vi "Example.vi"() -> ()   [LabVIEW 2019, in "BlueSerializationExample.lvlib"]
uses:
  BlueSerializationExample.lvlib
  BlueSerializable/BlueSerializable.lvclass
  BlueSerializer/BlueSerializer.lvclass
  2a9530f9-e359-4f49-87ca-caff470224ac.vi
  BlueSerializer/Deserialize.vi
panel:
  out "Data out":T1
  out "always true":bool
  out "Serialized Data 2":string
  out "error out":errorcluster
  out "Serialized Data 1":string
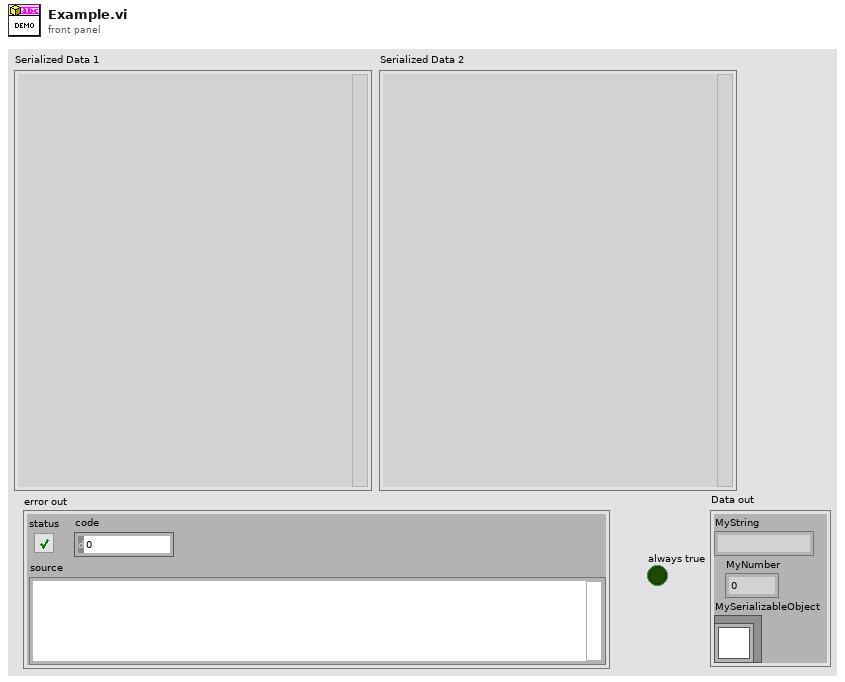
[diagram p1: front panel]
types:
  T1 = cluster{"MyString":string, "MyNumber":dbl, "MySerializableObject":refnum<class "BlueSerializable.lvclass">}
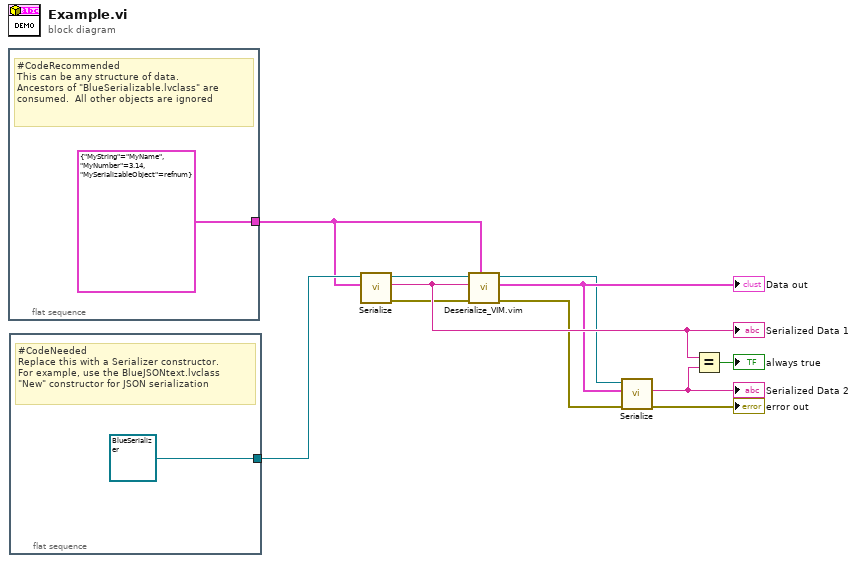
[diagram p0: block diagram]
diagram:
  n1 = flat-sequence {
    tunnel: [T1 {"MyString"="MyName", "MyNumber"=3.14, "MySerializableObject"=refnum}] -> w4
    frame #0 {
      # "#CodeRecommended\nThis can be any structure of data.\nAncestors of \"BlueSerializable.lvclass\" are consumed.  All other objects are ignored"
    }
  }
  n2 = flat-sequence {
    tunnel: [refnum<class "BlueSerializer.lvclass"> refnum ("BlueSerializer.lvlib:SerializerBase.lvclass")] -> w8
    frame #0 {
      # "#CodeNeeded\nReplace this with a Serializer constructor.\nFor example, use the BlueJSONtext.lvclass\n\"New\" constructor for JSON serialization"
    }
  }
  n3 = call "Serialize.vi"("Anything"=w4, "BlueSerializer in"=w8) -> ("error out"=w5:errorcluster, "Serialized Text"=w6:string, "BlueSerializer out"=w7:refnum<class "BlueSerializer.lvclass">)  [unwired: 7 in]
  "Serialized Data 1" <- w6
  n4 = call "Deserialize_VIM.vim"("Anything"=w4, "error in (no error)"=w5, "Serialized Text"=w6, "BlueSerializer in"=w7) -> ("error out"=w3:errorcluster, "Data out"=w2:T1, "BlueSerializer out"=w1:refnum<class "BlueSerializer.lvclass">)  [unwired: 5 in]
  "Data out" <- w2
  n5 = call "Serialize.vi"("error in (no error)"=w3, "Anything"=w2, "BlueSerializer in"=w1) -> ("error out"=→"error out":errorcluster, "Serialized Text"=w10:string)  [unwired: 6 in, 1 out]
  "Serialized Data 2" <- w10
  n6 = Equal?(x=w6, y=w10) -> (x = y?=→"always true":bool)
